vi "Read intDelay.vi"(8 "error in (no error)":errorcluster, 11 "CaptureSpectImage in":refnum<class "captureSpectImage.lvclass">) -> (0 "error out":errorcluster, 2 "intDelay":dbl, 3 "CaptureSpectImage out":refnum<class "captureSpectImage.lvclass">)   [LabVIEW 2016, in "Commands.lvlib" / "captureSpectImage.lvclass"]
uses:
  captureSpectImage.lvclass
  captureSpectImage.lvclass/captureSpectImage.ctl
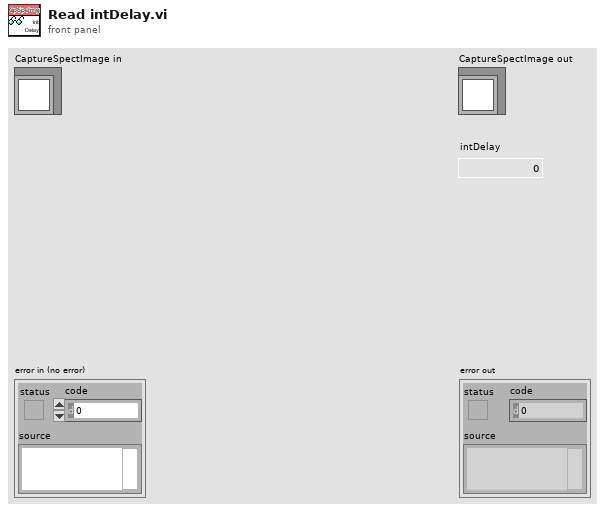
[diagram p1: front panel]
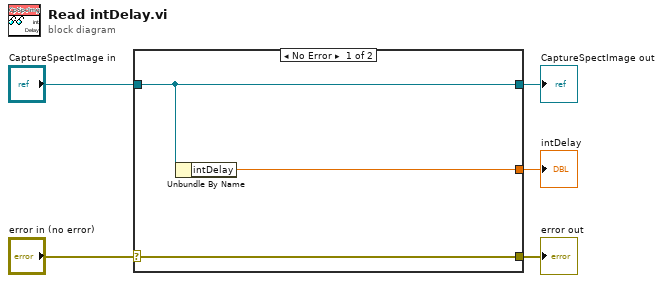
[diagram p0: block diagram]
diagram:
  n1 = case shown="No Error" "error in (no error)" {
    selector: "error in (no error)" -> [w8 w9]
    tunnel: [w8 w9] -> w4
    tunnel: [w7 w10] -> w2
    tunnel: "CaptureSpectImage in" -> [w7 w10]
    tunnel: [w6 _] -> w1
    frame No Error {
      n2 = Unbundle By Name(w7) -> ("intDelay"=w6:dbl)
    }
    frame Error {
    }
  }
  "error out" <- w4
  "CaptureSpectImage out" <- w2
  "intDelay" <- w1
